vi "UDP_Basic_Server.vi"(3 "error In":errorcluster, 4 "Data in":variant, 6 "Connection ID":refnum<k16>) -> (0 "warning out":errorcluster, 2 "Connection ID out":refnum<k16>)   [LabVIEW 2010]
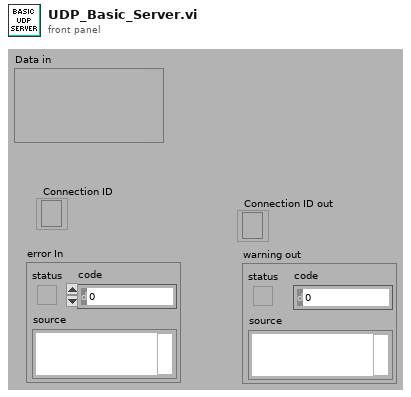
[diagram p1: front panel]
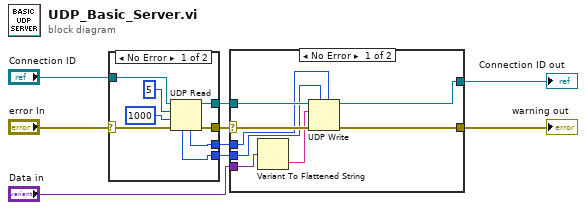
[diagram p0: block diagram]
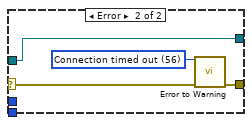
[diagram p2: hidden frame]
diagram:
  n1 = case shown="No Error" "error In" {
    selector: "error In" -> [w15 w18]
    tunnel: "Connection ID" -> [w17 w19]
    tunnel: [w14 w19] -> w4
    tunnel: [w13 w18] -> w8
    tunnel: [w11 _] -> w6
    tunnel: [w12 _] -> w5
    frame No Error {
      n2 = UDP Read(connection ID=w17, max size (548)=5, timeout ms (25000)=1000, 8:w15) -> (error out=w13:errorcluster, 3:w14:refnum<k16>, 4:w11:u16, 6:w12:u32)  [unwired: 1 out]
    }
    frame Error {
    }
  }
  n3 = case shown="No Error" w8 {
    selector: w8 -> [w27 w29]
    tunnel: w4 -> [w24 w31]
    tunnel: [w26 w28] -> w7
    tunnel: [w25 w31] -> w1
    tunnel: w5 -> [w22 _]
    tunnel: w6 -> [w23 _]
    tunnel: "Data in" -> [w20 _]
    frame No Error {
      n4 = Variant To Flattened String(Variant=w20) -> (data string=w21:string)  [unwired: 1 out]
      n5 = UDP Write(address=w22, port or service name=w23, connection ID=w24, data in=w21, 8:w27) -> (error out=w26:errorcluster, 3:w25:refnum<k16>)  [unwired: 1 in]
    }
    frame Error {
      w30 = 56 items=["No Error", "Argument Error", "Memory Full", "Out of Zone", "End of File", "File Already Open", "Generic File IO Error", "File Not Found", "File Permission Error", "Disk Full", "Duplicate Path", "Too Many Files Open", "Not Enabled", "Resource File Not Found", "Cannot Add Resource", "Resource Not Found", "Image Not Found", "Image Memory Error", "Pen Does Not Exist", "Config Bad Type", "Config Token Not Found", "Config Parse Error", "Config Memory Error", "Bad External Code Format", "Bad External Code Offset", "External Code Not Present", "Null Window", "Destroy Window Mixup", "Null Menu", "Print Aborted", "Bad Print Record", "Print Driver Error", "Windows Error During Print", "Memory Error During Print", "Print Dialog Error", "Generic Print Error", "Invalid Device Refnum", "Device Not Found", "Device Parameter Error", "Device Unit Error", "Can't Open Device", "Device Call Aborted", "Generic Error", "Cancelled By User", "Object ID Too Low", "Object ID Too High", "Object Not In Heap", "Unknown Heap", "Bad DefProc ID", "DefProc Not In Table", "Message Out Of Range", "Null Method", "Unknown Message", "Manager Call Not Supported", "Bad address", "Connection In progress", "Connection timed out", "Connection is already in progress", "Network attribute not supported", "Network error", "Address in use", "System out of memory", "Connection aborted", "Connection refused", "Connection is not connected", "Connection is already connected", "Connection closed", "Initialize error (interapplication manager)", "Bad occurrence", "Wait on unbound occurrence handler", "Occurrence queue overflow", "Bad path", "Semaphore not signaled", "Unrecognized type (interapplication manager)"] ("1st Error to Convert")
      n6 = call <vilib>:"Error to Warning.vi"("1st Error to Convert"=w30, "error in"=w29) -> ("warning out"=w28:errorcluster)  [unwired: 13 in]
    }
  }
  "warning out" <- w7
  "Connection ID out" <- w1
